vi "Begin.vi"(8 "error in (no error)":errorcluster, 11 "System Actor in":refnum<class "System Actor.lvclass">) -> (0 "error out":errorcluster, 3 "System Actor out":refnum<class "System Actor.lvclass">)   [LabVIEW 2014, in "Robot Actor Framework.lvlib" / "System Actor.lvlib" / "System Actor.lvclass"]
uses:
  System Actor.lvclass
  System Actor.lvclass/System Actor.ctl
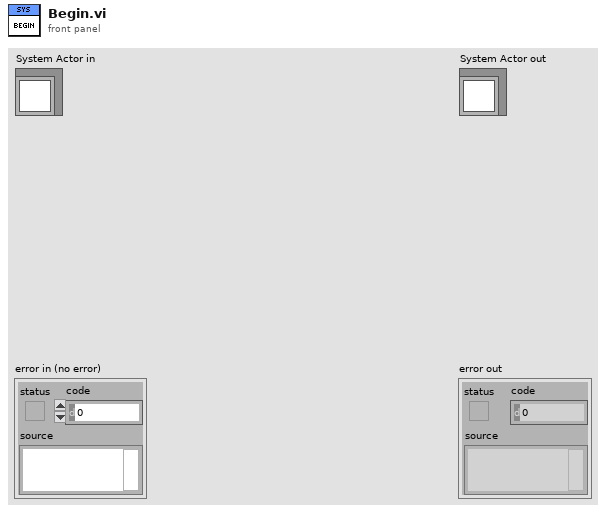
[diagram p1: front panel]
types:
  T1 = enum16{"Critical", "Error", "Warning", "Informational", "Debug"}
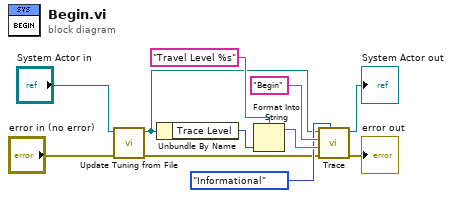
[diagram p0: block diagram]
diagram:
  n1 = call-dynamic "Update Tuning from File.vi"("error in (no error)"="error in (no error)", "System Actor in"="System Actor in") -> ("error out"=w1:errorcluster, "System Actor out"=w3:refnum<class "System Actor.lvclass">)  [unwired: 6 in, 2 out]
  n2 = Unbundle By Name(w3) -> ("Trace Level"=w10:T1)
  n3 = Format Into String(format string="Travel Level %s", w10) -> (resulting string=w8:string)  [unwired: 2 in, 1 out]
  n4 = call-dynamic "Trace.vi"("Trace Level"=T1."Informational", "error in (no error)"=w1, "System Message"=w8, "System Action"="Begin" ("Trace Message"), "System Actor in"=w3) -> ("error out"=→"error out":errorcluster, "System Actor out"=→"System Actor out":refnum<class "System Actor.lvclass">)  [unwired: 5 in]
